vi "subBuildTransferFunction.vi"(0 "PZarray":T1(array[cluster])) -> (7 "a":dbl[](array[numeric]), 8 "b":dbl[](array[numeric]))   [LabVIEW 2011]
uses:
  <vilib>/Analysis/2dsp.llb/1D Convolution (DBL).vi
  <vilib>/Analysis/NI_AALPro.lvlib
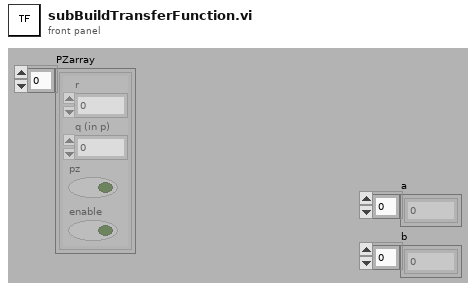
[diagram p1: front panel]
types:
  T1 = cluster{"r":dbl, "q (in p)":dbl, "pz":bool, "enable":bool}[]
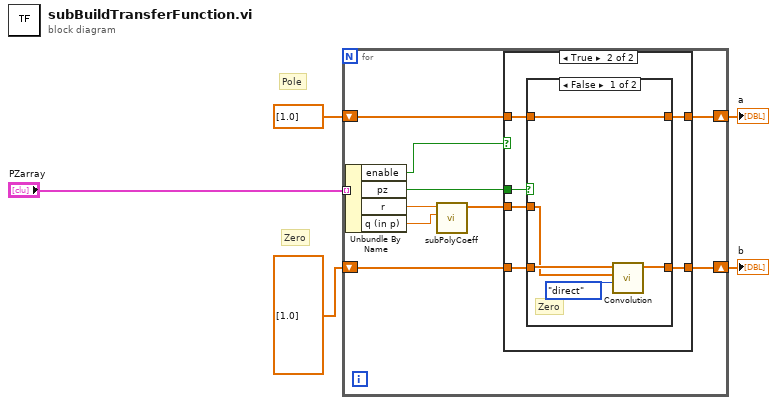
[diagram p0: block diagram]
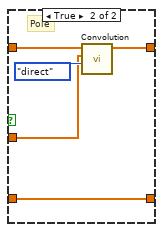
[diagram p3: hidden frame]
diagram:
  # "Zero"
  # "Pole"
  n1 = for {
    tunnel: "PZarray" -> [w15] mode=indexing
    shift-right: [w11] -> w3
    shift-left: dbl[] [1.0] -> [w13]
    shift-right: [w10] -> w2
    shift-left: dbl[] [1.0] -> [w12]
    n2 = Unbundle By Name(w15) -> ("enable"=w7:bool, "pz"=w6:bool, "r"=w9:dbl, "q (in p)"=w8:dbl)
    n3 = call "subPolyCoeff.vi"("theta"=w8, "r"=w9) -> ("Coeff"=w14:dbl[])  [unwired: 9 in]
    n4 = case shown="True" w7 {
      tunnel: w14 -> [_ w23]
      tunnel: w13 -> [w17 w22]
      tunnel: w12 -> [w16 w21]
      tunnel: [w17 w20] -> w11
      tunnel: [w16 w19] -> w10
      tunnel: w6 -> [_ w18]
      frame False {
      }
      frame True {
        n5 = case shown="False" w18 {
          tunnel: w23 -> [w24 w31]
          tunnel: w22 -> [w28 w32]
          tunnel: w21 -> [w25 w29]
          tunnel: [w28 w30] -> w20
          tunnel: [w26 w29] -> w19
          frame False {
            # "Zero"
            n6 = call-poly <vilib>:"Convolution.vi"("algorithm"=enum32{"direct", "frequency domain"}."direct", "Y"=w24, "X"=w25) -> ("X * Y"=w26:dbl[])  [unwired: 7 in, 1 out]
          }
          frame True {
            # "Pole"
            n7 = call-poly <vilib>:"Convolution.vi"("algorithm"=enum32{"direct", "frequency domain"}."direct", "Y"=w31, "X"=w32) -> ("X * Y"=w30:dbl[])  [unwired: 7 in, 1 out]
          }
        }
      }
    }
  }
  "a" <- w3
  "b" <- w2
